vi "Controller and 3D Model.vi"() -> ()   [LabVIEW 2012]
uses:
  <vilib>/Instr/_visa.llb/VISA Flush IO Buffer Mask.ctl
  <vilib>/Utility/miscctls.llb/LV3DPointTypeDef.ctl
  <vilib>/Instr/_visa.llb/VISA Configure Serial Port (Instr).vi
  <vilib>/picture/3D Picture Control/NI_3D Picture Control.lvlib
panel:
  out "X Chart 2":i32(graph)
  out "sum":i32
  out "x-y*floor(x/y)":i32
  out "Y Chart":i32(graph)
  out "X Chart":i32(graph)
  out "3D Picture Control":refnum<vi>(3d-picture)
  in  "STL File Path":path
  in  "Hexadecimal Input String":string
  in  "Stop":bool
  in  "UART configuration":enum32{"Basic", "Advanced"}(tab)
  in  "Port name":refnum<visa-resource-name>
  in  "Baud rate":T1(ring)
  in  "Data bits":u16=8 min=5 max=8 step=1
  in  "Stop bits":u16(ring)=10 items=["1.0"=10, "1.5"=15, "2.0"=20]
  in  "parity (0:none)":enum16{"None", "Odd", "Even", "Mark", "Space"}(ring)
  in  "Loop wait [ms]":u32
  in  "Waiting time [ms]":u32
  in  "Timeout [ms]":u32=10000
  in  "Flow control":u16(ring) items=["None", "XON/XOFF", "RTS/CTS", "XON/XOFF & RTS/CTS", "DTR/DSR", "XON/XOFF & DTR/DSR"]
  in  "Termination char\n(0xA = '\\n' = LF)":u8=10 format="%.0x"
  in  "Enable Termination\nChar (T)":bool=TRUE
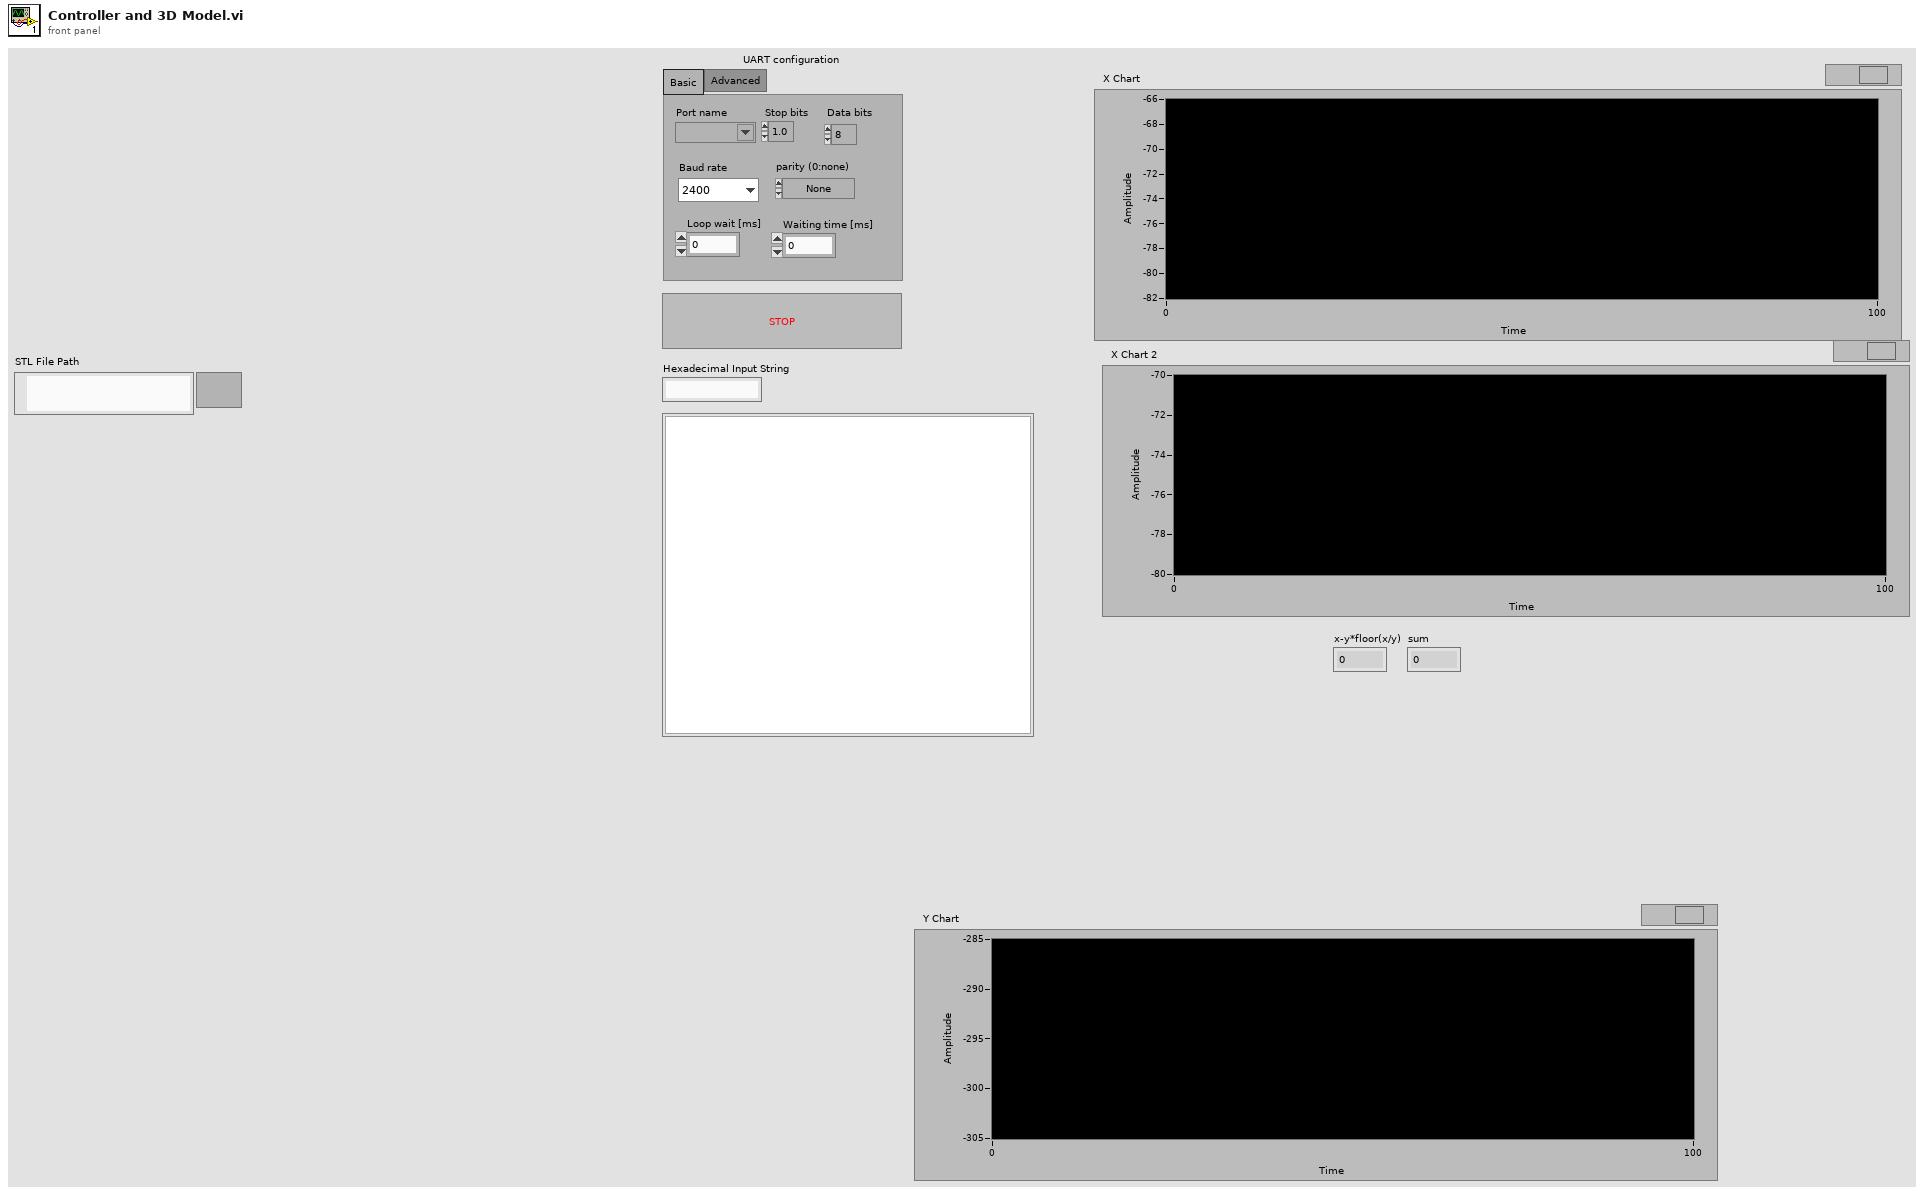
[diagram p1: front panel]
types:
  T1 = enum16{"2400\n", "4800", "9600\n", "19200", "38400", "57600", "115200"}
  T2 = typedef "LV3DPointTypeDef.ctl" = cluster{"X":sgl, "Y":sgl, "Z":sgl}
  T3 = typedef "VISA Flush IO Buffer Mask.ctl" = u16
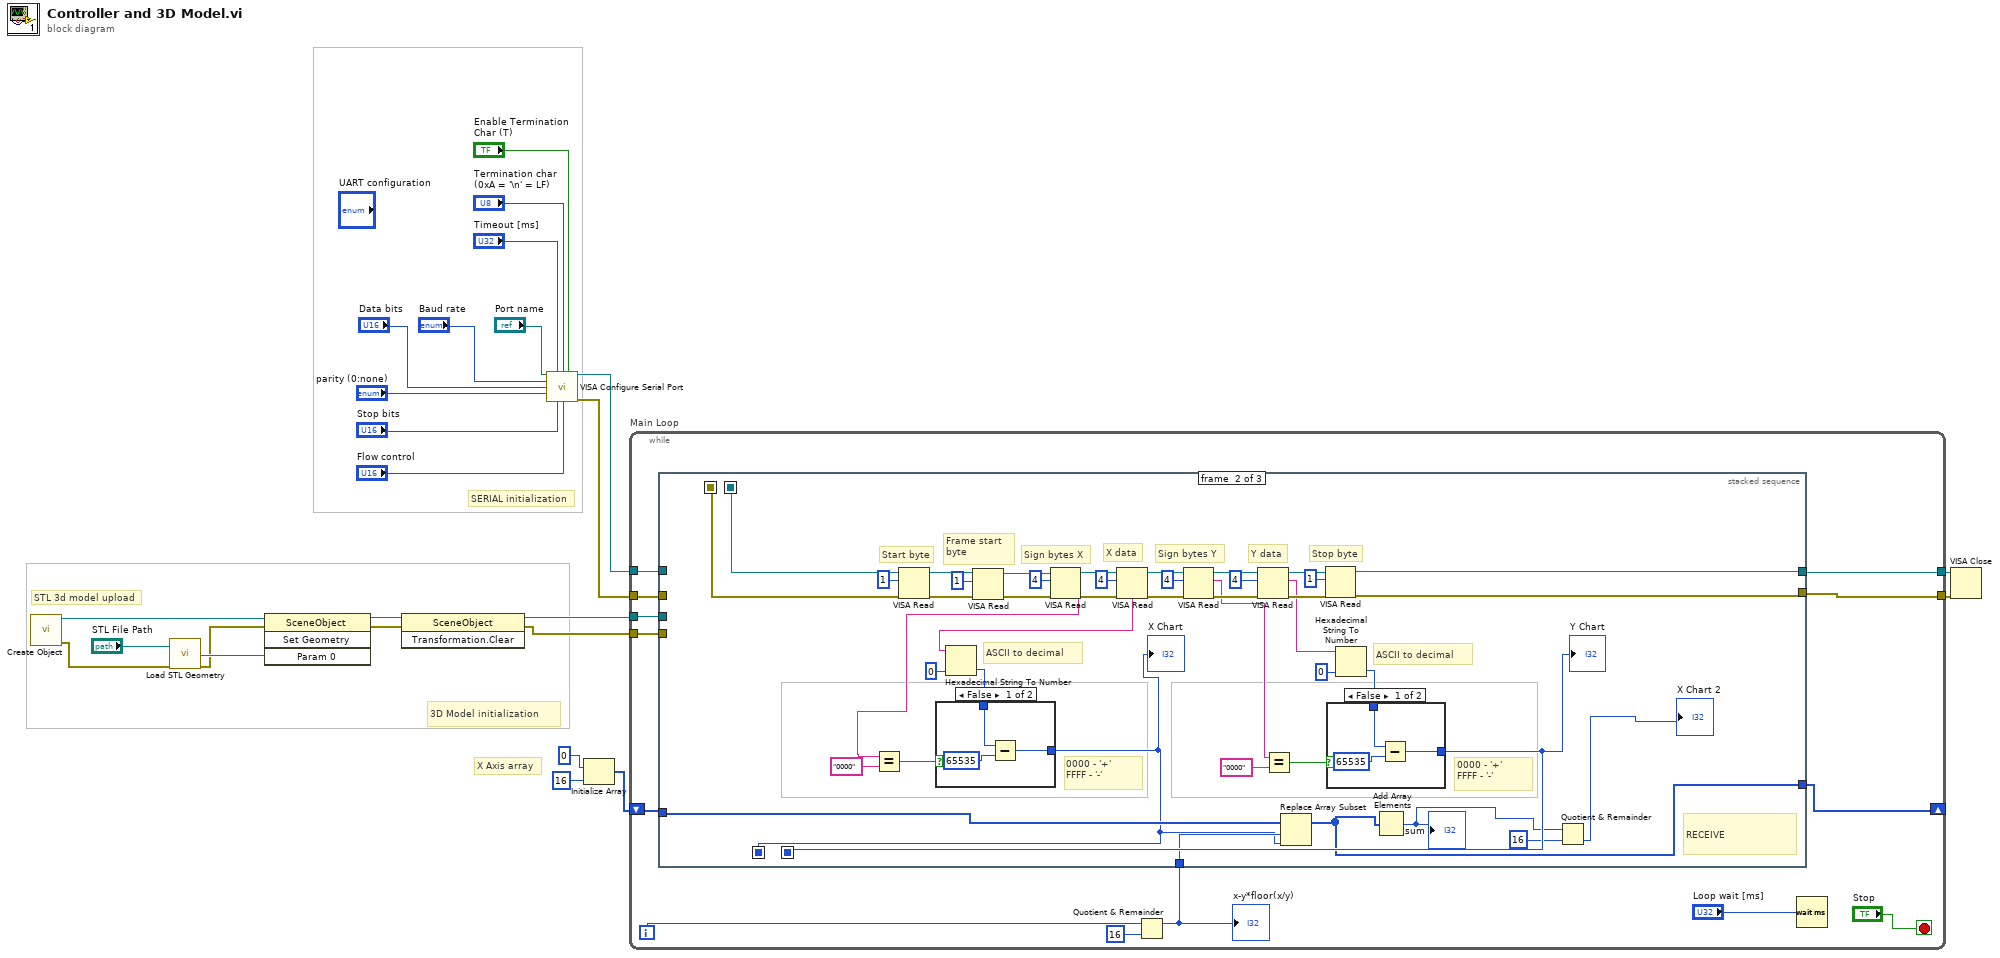
[diagram p0: block diagram]
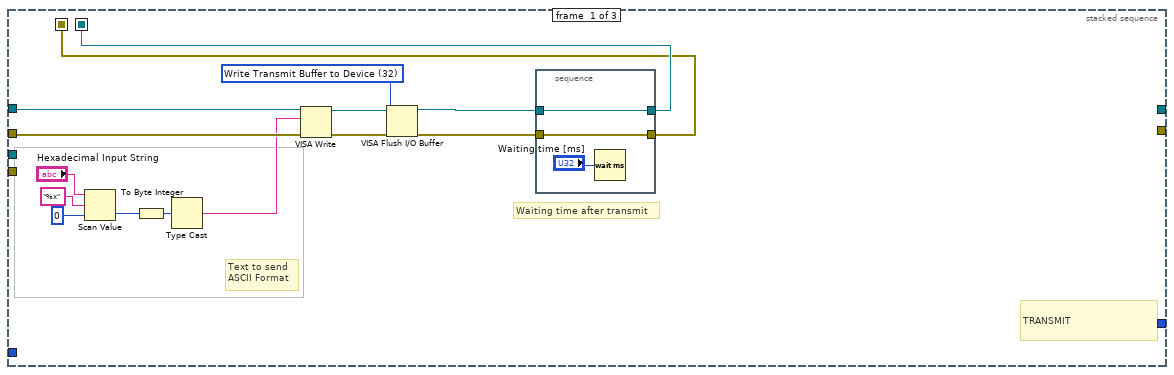
[diagram p2: hidden frame]
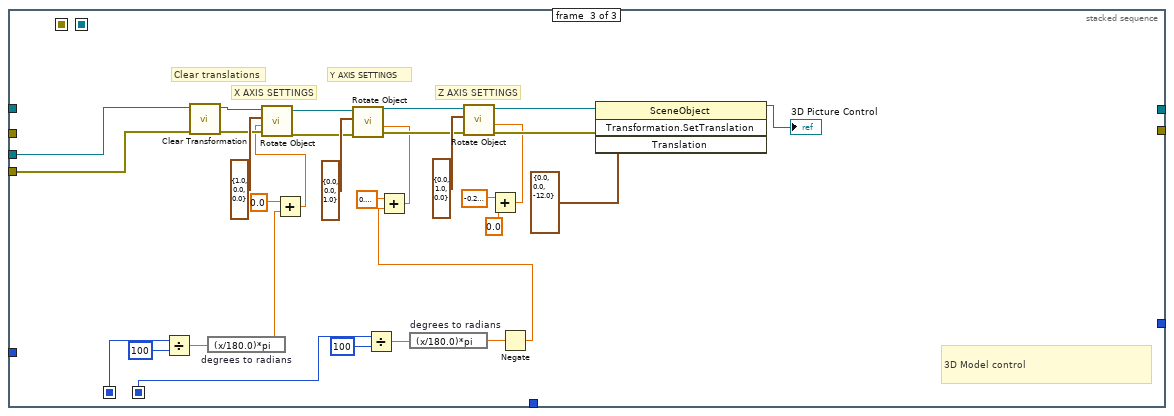
[diagram p5: hidden frame]
diagram:
  # "X Axis array"
  # "3D Model initialization"
  # "STL 3d model upload"
  # "SERIAL initialization"
  n1 = call <vilib>:"Create Object.vi"() -> ("error out"=w11:errorcluster, "Scene:New Object"=w9:refnum<vi>)  [unwired: 2 in, 8 out]
  n2 = call <vilib>:"Load STL Geometry.vi"("error in (no error)"=w11, "Model File"="STL File Path") -> ("error out"=w8:errorcluster, "New Mesh Refnum"=w10:refnum<vi>)  [unwired: 8 out]
  n3 = invoke class="SceneObject" method="Set Geometry"(reference=w9, error in=w8, "Param 0"=w10) -> (reference out=w7:refnum<vi>, error out=w6:errorcluster)  [unwired: 1 in, 2 out]
  n4 = invoke class="SceneObject" method="Transformation.Clear"(reference=w7, error in=w6) -> (reference out=w5:refnum<vi>, error out=w4:errorcluster)  [unwired: 1 in, 1 out]
  n5 = call-poly "VISA Configure Serial Port"("VISA resource name"="Port name", "timeout (10sec)"="Timeout [ms]", "termination char\n(0xA = '\\n' = LF)"="Termination char\n(0xA = '\\n' = LF)", "Enable Termination\nChar (T)"="Enable Termination\nChar (T)", "baud rate (9600)"="Baud rate", "data bits (8)"="Data bits", "parity (0:none)"="parity (0:none)", "stop bits (10: 1 bit)"="Stop bits", "flow control (0:none)"="Flow control") -> ("VISA resource name out"=w16:refnum<visa-resource-name>, "error out"=w15:errorcluster)  [unwired: 5 in]
  n6 = Initialize Array(0 ("element"), 16 ("dimension size")) -> (w1:i32[])
  n7 = while "Main Loop" {
    tunnel: w16 -> [w38]
    tunnel: w15 -> [w37]
    tunnel: [w33] -> w14
    tunnel: [w34] -> w13
    tunnel: w5 -> [w32]
    tunnel: w4 -> [w31]
    shift-right: [w27] -> _
    shift-left: w1 -> [w26]
    i -> [w30]
    stop <- "Stop" stop-if-true
    n8 = Quotient & Remainder(x=w30, y=16) -> (x-y*floor(x/y)=w28:i32)  [unwired: 1 out]
    "x-y*floor(x/y)" <- w28
    n9 = stacked-sequence "1 - Transmit, 2 - Receive" {
      seq-local: [w48 _ _] -> [_ w76 _]
      seq-local: [w47 _ _] -> [_ w77 _]
      seq-local: [_ w61 _] -> [_ _ w119]
      seq-local: [_ w64 _] -> [_ _ w110]
      tunnel: w38 -> [w50 _ _]
      tunnel: w37 -> [w49 _ _]
      tunnel: [_ w73 _] -> w34
      tunnel: [_ w72 _] -> w33
      tunnel: w32 -> [_ _ w116]
      tunnel: w31 -> [_ _ w115]
      tunnel: w26 -> [_ w63 _]
      tunnel: w28 -> [_ w62 _]
      tunnel: [_ w60 _] -> w27
      frame #0 {
        w51 = T3 32 items=["Flush Receive Buffer"=16, "Write Transmit Buffer to Device"=32, "Flush Receive Buffer (No I/O)"=64, "Flush Transmit Buffer"=128] ("Mask")
        # "TRANSMIT"
        # "Waiting time after transmit"
        # "Text to send\nASCII Format"
        n10 = Scan Value(string="Hexadecimal Input String", format string="%x", default (0 dbl)=0) -> (value=w42:i32)  [unwired: 1 out]
        n11 = To Byte Integer(number=w42) -> (8bit integer=w41:i8)
        n12 = Type Cast(x=w41) -> (*(type *) &x=w43:string)  [unwired: 1 in]
        n13 = VISA Write(VISA resource name=w50, write buffer=w43, error in (no error)=w49) -> (VISA resource name out=w52:refnum<visa-resource-name>, error out=w53:errorcluster)  [unwired: 1 out]
        n14 = VISA Flush I/O Buffer(VISA resource name=w52, mask (16)=w51, error in (no error)=w53) -> (VISA resource name out=w39:refnum<visa-resource-name>, error out=w40:errorcluster)
        n15 = stacked-sequence "Waiting time" {
          tunnel: [w55] -> w48
          tunnel: w39 -> [w55]
          tunnel: [w54] -> w47
          tunnel: w40 -> [w54]
          frame #0 {
            n16 = Wait (ms)(milliseconds to wait="Waiting time [ms]") -> ()  [unwired: 1 out]
          }
        }
      }
      frame #1 {
        # "0000 - '+'\nFFFF - '-'"
        # "ASCII to decimal"
        # "Stop byte"
        # "Y data"
        # "Sign bytes Y"
        # "RECEIVE"
        # "0000 - '+'\nFFFF - '-'"
        # "ASCII to decimal"
        # "X data"
        # "Sign bytes X"
        # "Frame start byte"
        # "Start byte"
        n17 = VISA Read(VISA resource name=w76, byte count=u32 1, error in (no error)=w77) -> (VISA resource name out=w98:refnum<visa-resource-name>, error out=w97:errorcluster)  [unwired: 2 out]
        n18 = VISA Read(VISA resource name=w98, byte count=u32 1, error in (no error)=w97) -> (VISA resource name out=w89:refnum<visa-resource-name>, error out=w85:errorcluster)  [unwired: 2 out]
        n19 = VISA Read(VISA resource name=w89, byte count=u32 4, error in (no error)=w85) -> (VISA resource name out=w88:refnum<visa-resource-name>, read buffer=w79:string, error out=w86:errorcluster)  [unwired: 1 out]
        n20 = Equal?(x=w79, y="0000") -> (x = y?=w78:bool)
        n21 = VISA Read(VISA resource name=w88, byte count=u32 4, error in (no error)=w86) -> (VISA resource name out=w95:refnum<visa-resource-name>, read buffer=w83:string, error out=w94:errorcluster)  [unwired: 1 out]
        n22 = Hexadecimal String To Number(string=w83, default (0uL)=0 ("default (0 U32)")) -> (number=w81:i32)  [unwired: 1 in, 1 out]
        n23 = case shown="False" w78 {
          tunnel: w81 -> [w105 w107]
          tunnel: [w106 w107] -> w61
          frame False {
            n24 = Subtract(x=w105, y=65535) -> (x-y=w106:i32)
          }
          frame True {
          }
        }
        "X Chart" <- w61
        n25 = VISA Read(VISA resource name=w95, byte count=u32 4, error in (no error)=w94) -> (VISA resource name out=w92:refnum<visa-resource-name>, read buffer=w65:string, error out=w91:errorcluster)  [unwired: 1 out]
        n26 = VISA Read(VISA resource name=w92, byte count=u32 4, error in (no error)=w91) -> (VISA resource name out=w75:refnum<visa-resource-name>, read buffer=w66:string, error out=w74:errorcluster)  [unwired: 1 out]
        n27 = Equal?(x=w65, y="0000") -> (x = y?=w67:bool)
        n28 = Replace Array Subset(array=w63, new element=w61, index=w62) -> (w60:i32[])
        n29 = VISA Read(VISA resource name=w75, byte count=u32 1, error in (no error)=w74) -> (VISA resource name out=w72:refnum<visa-resource-name>, error out=w73:errorcluster)  [unwired: 2 out]
        n30 = Hexadecimal String To Number(string=w66, default (0uL)=0 ("default (0 U32)")) -> (number=w69:i32)  [unwired: 1 in, 1 out]
        n31 = case shown="False" w67 {
          tunnel: w69 -> [w101 w103]
          tunnel: [w102 w103] -> w64
          frame False {
            n32 = Subtract(x=w101, y=65535) -> (x-y=w102:i32)
          }
          frame True {
          }
        }
        "Y Chart" <- w64
        n33 = Add Array Elements(numeric array=w60) -> (sum=w58:i32)
        "sum" <- w58
        n34 = Quotient & Remainder(x=w58, y=16) -> (floor(x/y)=→"X Chart 2":i32)  [unwired: 1 out]
      }
      frame #2 {
        # "3D Model control"
        # "Z AXIS SETTINGS"
        # "Y AXIS SETTINGS"
        # "Clear translations"
        # "X AXIS SETTINGS"
        n35 = Divide(x=w119, y=100) -> (x/y=w117:dbl)
        n36 = call <vilib>:"Clear Transformation.vi"("error in (no error)"=w115, "Object Refnum In"=w116) -> ("error out"=w127:errorcluster, "Object Refnum Out"=w137:refnum<vi>)  [unwired: 8 out]
        n37 = expression code="(x/180.0)*pi" "degrees to radians"(w117) -> (w113:dbl)
        n38 = Add(x=sgl 0.0 ("default X"), y=w113) -> (x+y=w125:dbl)
        n39 = call <vilib>:"Rotate Object.vi"("error in (no error)"=w127, "Angle"=w125, "Axis"=cluster{"X":sgl, "Y":sgl, "Z":sgl} {"X"=1.0, "Y"=0.0, "Z"=0.0}, "Scene.Object In"=w137) -> ("error out"=w128:errorcluster, "Scene.Object Out"=w129:refnum<vi>)  [unwired: 6 out]
        n40 = Divide(x=w110, y=100) -> (x/y=w111:dbl)
        n41 = expression code="(x/180.0)*pi" "degrees to radians"(w111) -> (w109:dbl)
        n42 = Add(x=sgl -0.2 ("Z"), y=sgl 0.0) -> (x+y=w120:sgl)
        n43 = Negate(x=w109) -> (-x=w108:dbl)
        n44 = Add(x=sgl 0.6 ("default Y"), y=w108) -> (x+y=w122:dbl)
        n45 = call <vilib>:"Rotate Object.vi"("error in (no error)"=w128, "Angle"=w122, "Axis"=cluster{"X":sgl, "Y":sgl, "Z":sgl} {"X"=0.0, "Y"=0.0, "Z"=1.0}, "Scene.Object In"=w129) -> ("error out"=w130:errorcluster, "Scene.Object Out"=w131:refnum<vi>)  [unwired: 6 out]
        n46 = call <vilib>:"Rotate Object.vi"("error in (no error)"=w130, "Angle"=w120, "Axis"=cluster{"X":sgl, "Y":sgl, "Z":sgl} {"X"=0.0, "Y"=1.0, "Z"=0.0}, "Scene.Object In"=w131) -> ("error out"=w132:errorcluster, "Scene.Object Out"=w133:refnum<vi>)  [unwired: 6 out]
        n47 = invoke class="SceneObject" method="Transformation.SetTranslation"(reference=w133, error in=w132, "Translation"=T2 {"X"=0.0, "Y"=0.0, "Z"=-12.0}) -> (reference out=→"3D Picture Control":refnum<vi>)  [unwired: 1 in, 3 out]
      }
    }
    n48 = Wait (ms)(milliseconds to wait="Loop wait [ms]") -> ()  [unwired: 1 out]
  }
  n49 = VISA Close(VISA resource name=w14, error in (no error)=w13) -> ()  [unwired: 1 out]
